vi "odd_even.vi"() -> ()   [LabVIEW 2020]
panel:
  out "ODD":bool
  out "EVEN":bool
  in  "A":dbl
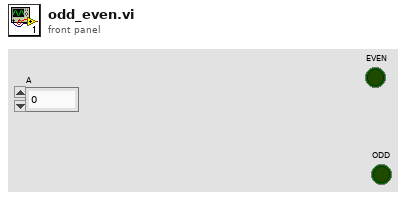
[diagram p1: front panel]
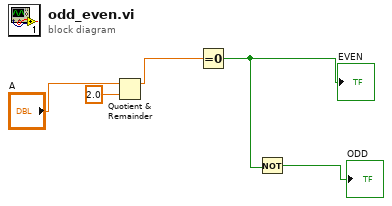
[diagram p0: block diagram]
diagram:
  n1 = Quotient & Remainder(x="A", y=2.0) -> (x-y*floor(x/y)=w3:dbl)  [unwired: 1 out]
  n2 = Equal To 0?(x=w3) -> (x = 0?=w2:bool)
  "EVEN" <- w2
  n3 = Not(x=w2) -> (.not. x?=→"ODD":bool)
